vi "get_communications_configuration.vi"(8 "error in (no error)":errorcluster, 10 "Comms":string(combo)="330", 11 "connection ID":refnum<k5>) -> (0 "error out":errorcluster, 2 "Comms configuration cluster":T1, 3 "connection ID out":refnum<k5>)   [LabVIEW 2018]
uses:
  typedefs/communications_configuration.ctl
panel:
  in  "Separation char (Omega protocol, continuous data mode)":string(combo)="0"
  in  "Response echo enabled":string(combo)="0"
  in  "Line feed enabled":string(combo)="0"
  in  "Data mode":string(combo)="0"
  in  "Protocol":string(combo)="0"
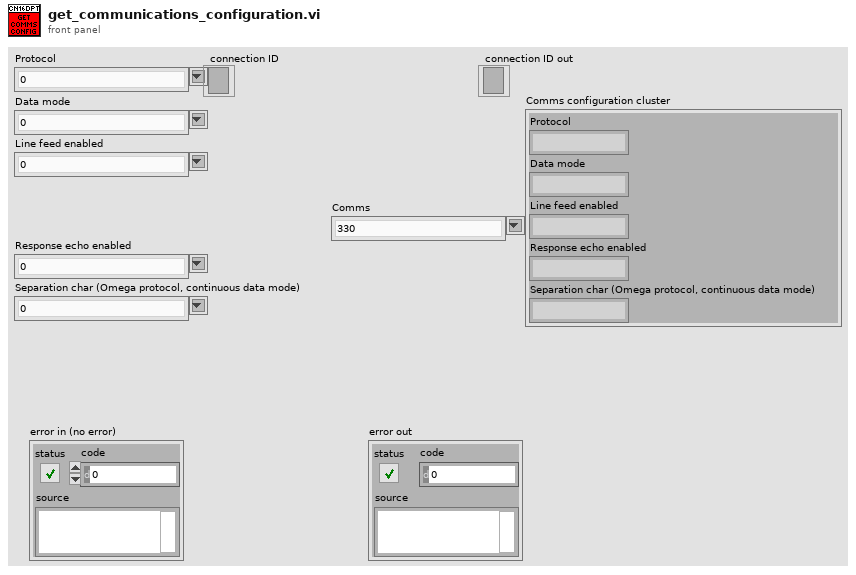
[diagram p1: front panel]
types:
  T1 = typedef "communications_configuration.ctl" = cluster{"Protocol":string, "Data mode":string, "Line feed enabled":string, "Response echo enabled":string, "Separation char (Omega protocol, continuous data mode)":string}
  T2 = typedef "LVComboBoxStrsAndValuesArrayTypeDef.ctl" = cluster{"String":string, "Value":string}[]
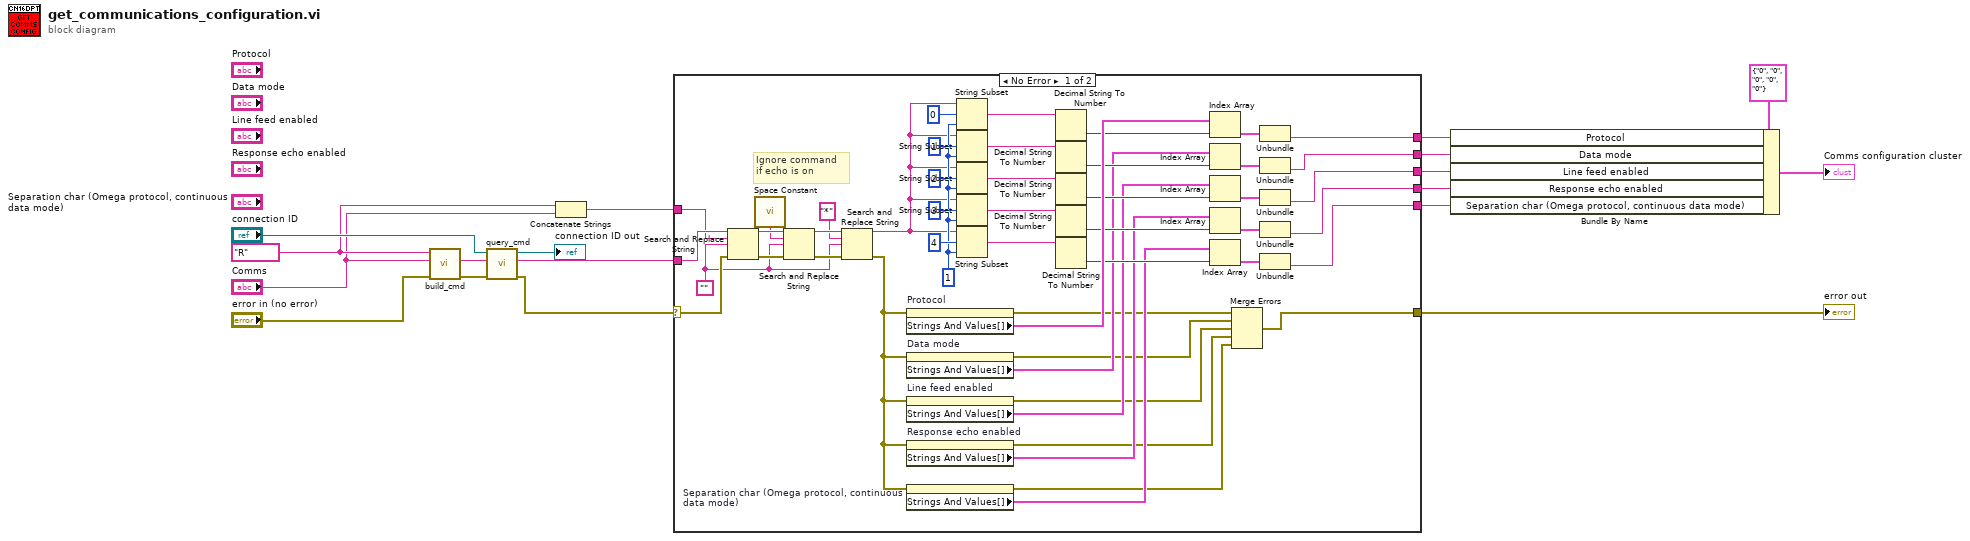
[diagram p0: block diagram]
diagram:
  w6 = "R" ("Command class")
  n1 = call "build_cmd.vi"("error in (no error)"="error in (no error)", "Command ID"="Comms", "Command class"=w6) -> ("error out"=w17:errorcluster, "Command"=w16:string)  [unwired: 7 in]
  n2 = call "query_cmd.vi"("error in (no error)"=w17, "Command"=w16, "connection ID"="connection ID") -> ("error out"=w12:errorcluster, "Response"=w13:string, "connection ID out"=→"connection ID out":refnum<k5>)  [unwired: 6 in]
  n3 = Concatenate Strings(w6, "Comms") -> (w4:string)
  n4 = case shown="No Error" w12 {
    selector: w12 -> [w38 w68]
    tunnel: w13 -> [w40 _]
    tunnel: [w27 _] -> w11
    tunnel: [w22 _] -> w10
    tunnel: [w21 _] -> w9
    tunnel: [w20 _] -> w8
    tunnel: [w19 _] -> w7
    tunnel: [w41 w68] -> w1
    tunnel: w4 -> [w39 _]
    frame No Error {
      w32 = ""
      w60 = 1 ("offset (0)")
      # "Ignore command\nif echo is on"
      n5 = Search and Replace String(input string=w40, search string=w39, replace string=w32, error in=w38) -> (result string=w37:string, error out=w36:errorcluster)  [unwired: 4 in, 2 out]
      n6 = call <vilib>:"Space Constant.vi"() -> ("String"=w35:string)
      n7 = Search and Replace String(input string=w37, search string=w35, replace string=w32, error in=w36) -> (result string=w34:string, error out=w33:errorcluster)  [unwired: 4 in, 2 out]
      n8 = Search and Replace String(input string=w34, search string="*", replace string=w32, error in=w33) -> (result string=w29:string, error out=w30:errorcluster)  [unwired: 4 in, 2 out]
      n9 = property on="Protocol" class="CmbBox"(error in=w30) -> (error out=w46:errorcluster, "Strings And Values[]"=w67:T2)  [unwired: 1 in, 1 out]
      n10 = property on="Data mode" class="CmbBox"(error in=w30) -> (error out=w45:errorcluster, "Strings And Values[]"=w53:T2)  [unwired: 1 in, 1 out]
      n11 = property on="Line feed enabled" class="CmbBox"(error in=w30) -> (error out=w44:errorcluster, "Strings And Values[]"=w54:T2)  [unwired: 1 in, 1 out]
      n12 = property on="Response echo enabled" class="CmbBox"(error in=w30) -> (error out=w43:errorcluster, "Strings And Values[]"=w48:T2)  [unwired: 1 in, 1 out]
      n13 = property on="Separation char (Omega protocol, continuous data mode)" class="CmbBox"(error in=w30) -> (error out=w42:errorcluster, "Strings And Values[]"=w47:T2)  [unwired: 1 in, 1 out]
      n14 = String Subset(string=w29, offset (0)=0, length (rest)=w60) -> (substring=w59:string)
      n15 = String Subset(string=w29, offset (0)=1, length (rest)=w60) -> (substring=w52:string)
      n16 = String Subset(string=w29, offset (0)=2, length (rest)=w60) -> (substring=w51:string)
      n17 = String Subset(string=w29, offset (0)=3, length (rest)=w60) -> (substring=w50:string)
      n18 = String Subset(string=w29, offset (0)=4, length (rest)=w60) -> (substring=w49:string)
      n19 = Decimal String To Number(string=w59) -> (number=w66:i32)  [unwired: 2 in, 1 out]
      n20 = Decimal String To Number(string=w52) -> (number=w58:i32)  [unwired: 2 in, 1 out]
      n21 = Decimal String To Number(string=w51) -> (number=w57:i32)  [unwired: 2 in, 1 out]
      n22 = Decimal String To Number(string=w50) -> (number=w56:i32)  [unwired: 2 in, 1 out]
      n23 = Decimal String To Number(string=w49) -> (number=w55:i32)  [unwired: 2 in, 1 out]
      n24 = Index Array(array=w67, index=w66) -> (element=w28:cluster{"String":string, "Value":string})
      n25 = Index Array(array=w53, index=w58) -> (element=w26:cluster{"String":string, "Value":string})
      n26 = Index Array(array=w54, index=w57) -> (element=w25:cluster{"String":string, "Value":string})
      n27 = Index Array(array=w48, index=w56) -> (element=w24:cluster{"String":string, "Value":string})
      n28 = Index Array(array=w47, index=w55) -> (element=w23:cluster{"String":string, "Value":string})
      n29 = Merge Errors(w46, w45, w44, w43, w42) -> (w41:errorcluster)
      n30 = Unbundle(w28) -> ("Value"=w27:string)  [unwired: 1 out]
      n31 = Unbundle(w26) -> ("Value"=w22:string)  [unwired: 1 out]
      n32 = Unbundle(w25) -> ("Value"=w21:string)  [unwired: 1 out]
      n33 = Unbundle(w24) -> ("Value"=w20:string)  [unwired: 1 out]
      n34 = Unbundle(w23) -> ("Value"=w19:string)  [unwired: 1 out]
    }
    frame Error {
    }
  }
  "error out" <- w1
  n35 = Bundle By Name(cluster=T1 {"Protocol"="0", "Data mode"="0", "Line feed enabled"="0", "Response echo enabled"="0", "Separation char (Omega protocol, continuous data mode)"="0"} ("Comms configuration cluster"), "Protocol"=w11, "Data mode"=w10, "Line feed enabled"=w9, "Response echo enabled"=w8, "Separation char (Omega protocol, continuous data mode)"=w7) -> (→"Comms configuration cluster":T1)
